vi "File.Remove double backslashes from path.vi"(11 "Path":path) -> (3 "Path Out":path)   [LabVIEW 2018]
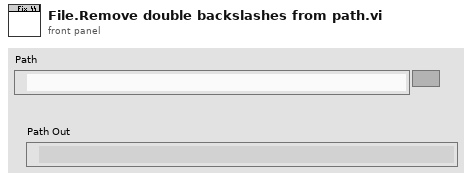
[diagram p1: front panel]
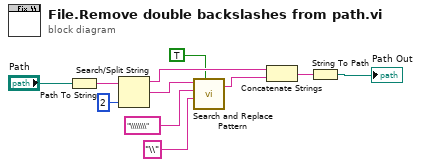
[diagram p0: block diagram]
diagram:
  n1 = Path To String(path="Path") -> (string=w11:string)
  n2 = Search/Split String(string=w11, offset (0)=2) -> (substring before match=w8:string, match + rest of string=w9:string)  [unwired: 1 in, 1 out]
  n3 = call <vilib>:"Search and Replace Pattern.vi"("string"=w9, "regular expression (\"\")"="\\\\\\\\" ("regular expression (\"\")"), "replace string (\"\")"="\\" ("regular expression (\"\")"), "replace all? (F)"=TRUE) -> ("result string"=w7:string)  [unwired: 1 in, 1 out]
  n4 = Concatenate Strings(w8, w7) -> (w4:string)
  n5 = String To Path(string=w4) -> (path=→"Path Out":path)
